vi "Label Targets.vi"(8 "Score Limit":dbl=75.0, 10 "Target Info":T3, 11 "Image in":T1) -> (3 "Image out":T1)   [LabVIEW 2025]
doc: "Draw text scores near or on the particle."
uses:
  TargetType.ctl
  <vilib>/vision/Image Controls.llb/IMAQ Image.ctl
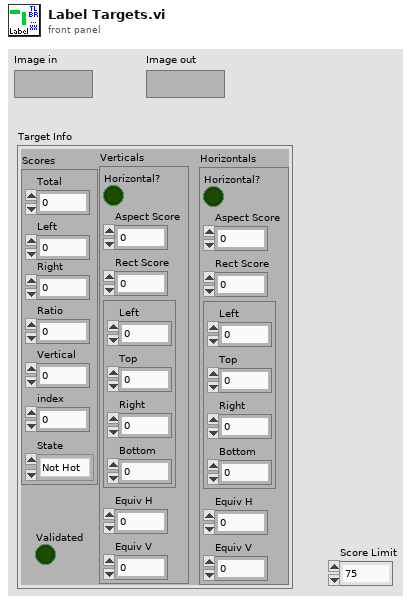
[diagram p1: front panel]
types:
  T1 = typedef "IMAQ Image.ctl" = refnum<image>
  T2 = typedef "TargetType.ctl" = enum16{"Not Hot", "Hot"}
  T3 = cluster{"Scores":cluster{"Total":dbl, "Left":dbl, "Right":dbl, "Ratio":dbl, "Vertical":dbl, "index":i32, "State":T2}, "Verticals":cluster{"Horizontal?":bool, "Aspect Score":dbl, "Rect Score":dbl, cluster{"Left":dbl, "Top":dbl, "Right":dbl, "Bottom":dbl}, "Equiv H":dbl, "Equiv V":dbl}, "Horizontals":cluster{"Horizontal?":bool, "Aspect Score":dbl, "Rect Score":dbl, cluster{"Left":dbl, "Top":dbl, "Right":dbl, "Bottom":dbl}, "Equiv H":dbl, "Equiv V":dbl}, "Validated":bool}
  T4 = cluster{"Total":dbl, "Left":dbl, "Right":dbl, "Ratio":dbl, "Vertical":dbl, "index":i32, "State":T2}
  T5 = cluster{"Horizontal?":bool, "Aspect Score":dbl, "Rect Score":dbl, cluster{"Left":dbl, "Top":dbl, "Right":dbl, "Bottom":dbl}, "Equiv H":dbl, "Equiv V":dbl}
  T6 = cluster{"Left":dbl, "Top":dbl, "Right":dbl, "Bottom":dbl}
  T7 = cluster{"Left":dbl, "Right":dbl, "Ratio":dbl, "Vertical":dbl}
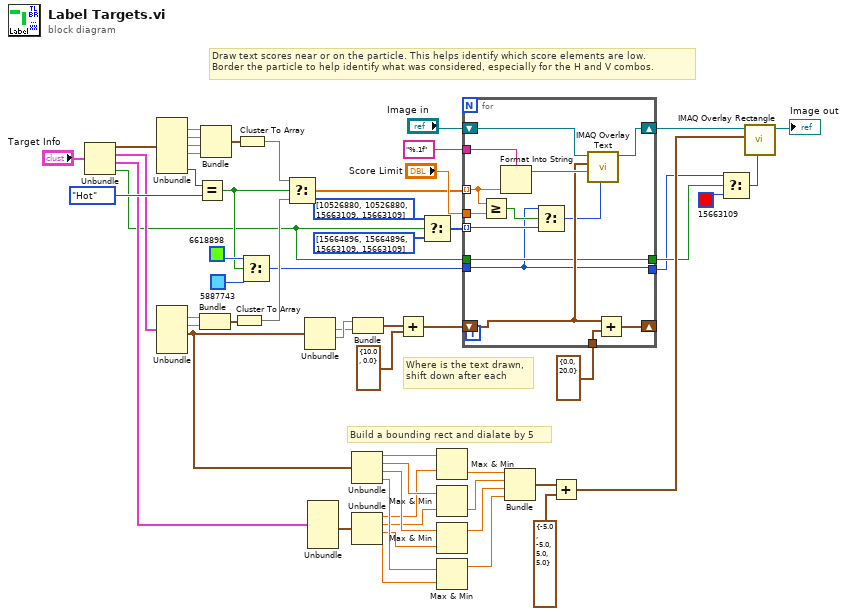
[diagram p0: block diagram]
diagram:
  # "Where is the text drawn,\nshift down after each"
  # "Build a bounding rect and dialate by 5"
  # "Draw text scores near or on the particle. This helps identify which score elements are low.\nBorder the particle to help identify what was considered, especially for the H and V combos."
  n1 = Unbundle("Target Info") -> ("Scores"=w42:T4, "Verticals"=w38:T5, "Horizontals"=w22:T5, "Validated"=w3:bool)
  n2 = Unbundle(w42) -> ("Left"=w53:dbl, "Right"=w50:dbl, "Ratio"=w51:dbl, "Vertical"=w52:dbl, "State"=w19:T2)  [unwired: 2 out]
  n3 = Unbundle(w38) -> ("Aspect Score"=w18:dbl, "Rect Score"=w17:dbl, w21:T6)  [unwired: 3 out]
  n4 = Equal?(x=w19, y=TargetType."Hot" ("State")) -> (x = y?=w5:bool)
  n5 = Bundle("Aspect Score"=w18, "Rect Score"=w17) -> (w16:cluster{"Aspect Score":dbl, "Rect Score":dbl})  [unwired: 1 in]
  n6 = Bundle("Left"=w53, "Right"=w50, "Ratio"=w51, "Vertical"=w52) -> (w49:T7)  [unwired: 1 in]
  n7 = Cluster To Array(cluster=w16) -> (array=w15:dbl[])
  n8 = Cluster To Array(cluster=w49) -> (array=w14:dbl[])
  n9 = Select(t=u32 6618898 ("Color"), s=w5, f=u32 5887743 ("Color")) -> (s? t:f=w4:u32)
  n10 = Select(t=w14, s=w5, f=w15) -> (s? t:f=w13:dbl[])
  n11 = Unbundle(w21) -> ("Top"=w40:dbl, "Right"=w41:dbl)  [unwired: 2 out]
  n12 = Unbundle(w22) -> (w24:T6)  [unwired: 5 out]
  n13 = Unbundle(w21) -> ("Left"=w25:dbl, "Top"=w27:dbl, "Right"=w29:dbl, "Bottom"=w31:dbl)
  n14 = Unbundle(w24) -> ("Left"=w26:dbl, "Top"=w28:dbl, "Right"=w30:dbl, "Bottom"=w32:dbl)
  n15 = Bundle("Right"=w41, "Top"=w40) -> (w39:cluster{"Right":dbl, "Top":dbl})  [unwired: 1 in]
  n16 = Add(x=w39, y=cluster{dbl, dbl} {10.0, 0.0} ("x+y")) -> (x+y=w55:cluster{dbl, dbl})
  n17 = Select(t=u32[] [10526880, 10526880, 15663109, 15663109], s=w3, f=u32[] [15664896, 15664896, 15663109, 15663109]) -> (s? t:f=w12:u32[])
  n18 = Max & Min(x=w25, y=w26) -> (min(x,y)=w33:dbl)  [unwired: 1 out]
  n19 = Max & Min(x=w27, y=w28) -> (min(x,y)=w34:dbl)  [unwired: 1 out]
  n20 = Max & Min(x=w29, y=w30) -> (max(x,y)=w35:dbl)  [unwired: 1 out]
  n21 = Max & Min(x=w31, y=w32) -> (max(x,y)=w36:dbl)  [unwired: 1 out]
  n22 = for {
    tunnel: w13 -> [w65] mode=indexing
    shift-right: [w68] -> _
    shift-left: w55 -> [w67]
    shift-right: [w69] -> w47
    shift-left: "Image in" -> [w70]
    tunnel: w12 -> [w66] mode=indexing
    tunnel: "Score Limit" -> [w64]
    tunnel: cluster{dbl, dbl} {0.0, 20.0} ("x+y") -> [w61]
    tunnel: "%.1f" ("format string") -> [w60]
    tunnel: w4 -> [w58]
    tunnel: w3 -> [w59]
    tunnel: [w59] -> w2
    tunnel: [w58] -> w1
    n23 = Greater Or Equal?(x=w65, y=w64) -> (x >= y?=w63:bool)
    n24 = Format Into String(format string=w60, w65) -> (resulting string=w71:string)  [unwired: 2 in, 1 out]
    n25 = Select(t=w58, s=w63, f=w66) -> (s? t:f=w62:u32)
    n26 = call "IMAQ Overlay Text"("Text Color (black)"=w62, "String"=w71, "Origin"=w67, "Image"=w70) -> ("Image Out"=w69:T1)  [unwired: 6 in, 1 out]
    n27 = Add(x=w61, y=w67) -> (x+y=w68:cluster{dbl, dbl})
  }
  n28 = Bundle(w33, w34, w35, w36) -> (w37:cluster{dbl, dbl, dbl, dbl})  [unwired: 1 in]
  n29 = Add(x=w37, y=cluster{dbl, dbl, dbl, dbl} {-5.0, -5.0, 5.0, 5.0} ("output cluster")) -> (x+y=w20:cluster{dbl, dbl, dbl, dbl})
  n30 = Select(t=w1, s=w2, f=u32 15663109 ("Color")) -> (s? t:f=w44:u32)
  n31 = call "IMAQ Overlay Rectangle"("Color"=w44, "Rectangle"=w20, "Image"=w47) -> ("Image Out"=→"Image out":T1)  [unwired: 7 in, 1 out]
